vi "File_Name_Append_Suffix.vi"(6 "New File Extension":string, 9 "Suffix":string, 10 "Rel_Path":path, 11 "Dest":path) -> (3 "Dest Path":path)   [LabVIEW 2020]
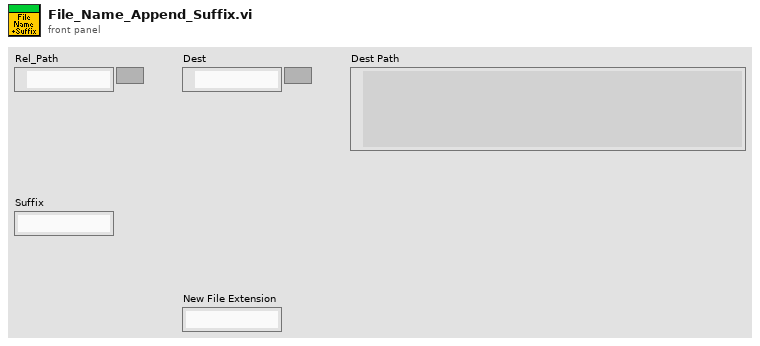
[diagram p1: front panel]
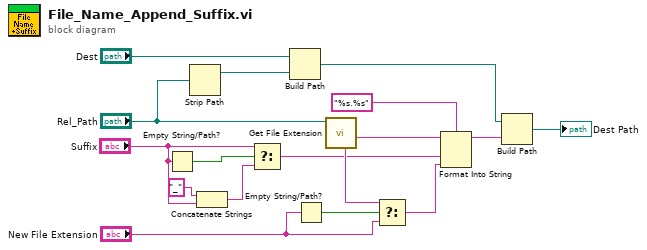
[diagram p0: block diagram]
diagram:
  n1 = Empty String/Path?(string/path="Suffix") -> (empty?=w9:bool)
  n2 = Strip Path(path="Rel_Path") -> (stripped path=w1:path)  [unwired: 1 out]
  n3 = Concatenate Strings("_" ("string"), "Suffix") -> (w8:string)
  n4 = Select(t="Suffix", s=w9, f=w8) -> (s? t:f=w5:string)
  n5 = Build Path(base path="Dest", name or relative path=w1) -> (appended path=w2:path)
  n6 = Empty String/Path?(string/path="New File Extension") -> (empty?=w11:bool)
  n7 = call <vilib>:"Get File Extension.vi"("file"="Rel_Path") -> ("filename without extension"=w13:string, "unmodified file extension"=w15:string)  [unwired: 6 in, 3 out]
  n8 = Select(t=w15, s=w11, f="New File Extension") -> (s? t:f=w12:string)
  n9 = Format Into String(format string="%s.%s", initial string=w13, w5, w12) -> (resulting string=w16:string)  [unwired: 1 in, 1 out]
  n10 = Build Path(base path=w2, name or relative path=w16) -> (appended path=→"Dest Path":path)
